vi "GoalieOld.vi"(6 "Defensores":u32[](array[numeric]), 7 "AI Parameters":T1={"GotoKick"={"Dist do cone a frente"=0.0, "attacker farback"=1000.0, "Perto"=300.0, "min dist to kick"=0.0, "kick eps"=110.0, "Time to transition"=0.05}, "Attacker"={"CC chute"=0.09, "CC passe"=0.045, "Kick Force"=200.0, "D ball-robot Kick"=200.0, "D ball-robot Pass"=0.0}, "Defender"={"D max"=1700.0, "Vel p/ robô av"=1000.0, "Kick Force"=100.0, "D atk-def"=300.0, "D farback"=400.0}, "Timeout"={"Field/v in x"=6.0, "Dist Robots"=300, "Dist up in y"=300}, "Pose Striker"={"dist"=200.0, "Numeric"=-4.0, "dist 2"=200.0}, "Dist Stop"=300.0, "Distance when ball out"=200, "D central gap "=150.0, "T pass"=0.0, "Force ++"=0.0, "range kick"=0.0, "Chute alto"=TRUE, "Marcador novo"=TRUE} {"D central gap" format="%#_13g"; "Dist Stop" format="%#_13g"; "Pose Striker"."Numeric" format="%#_13g"; "Defender"."Kick Force" format="%#_13g"; "Defender"."Vel p/ robô av" format="%#_13g"; "Attacker"."D ball-robot Kick" format="%#_13g"; "Attacker"."Kick Force" format="%#_13g"; "Attacker"."CC passe" format="%#_13g"; "Attacker"."CC chute" format="%#_13g"; "GotoKick"."min dist to kick" format="%#_13g"; "GotoKick"."Perto" format="%#_13g"; "GotoKick"."attacker farback" format="%#_13g"; "GotoKick"."Dist do cone a frente" format="%#_13g"}, 8 "Robot":T2={"id"=0, "function"=enum."Attacker", "x"=0.0, "y"=0.0, "orientation"=0.0, "v_tangent"=0.0, "v_normal"=0.0, "v_ang"=0.0, "kick_x"=0.0, "kick_z"=0.0, "dribble"=FALSE, "Timestamp"=timestamp(0 s since 1904-01-01), "estimatives"={"est_v_tangent"=0.0, "est_v_normal"=0.0, "est_vx"=0.0, "est_vy"=0.0, "Pos Robot Est"=[]}, "dest_x_kick"=0.0, "dest_y_kick"=0.0, "Gap Coord"=[], "States"=enum."GoToTangent", "Path "=[], "Path  Smooth"=[], "Dest"=[]}, 10 "Field defense":dbl[](array[numeric]), 11 "IA Input":T7={"our_robots"=[], "enemy_robots"=[], "balls"=[], "geometry"={"line_width"=0, "field_length"=0, "field_width"=0, "boundary_width"=0, "referee_width"=0, "goal_width"=0, "goal_depth"=0, "goal_wall_width"=0, "center_circle_radius"=0, "defense_radius"=0, "defense_stretch"=0, "free_kick_from_defense_dist"=0, "penalty_spot_from_field_line_dist"=0, "penalty_line_from_spot_dist"=0}, "IA Judge"={"stage"="", "command"="", "our_goalie_id"=0.0, "enemy_goalie_id"=0.0, "command enum"=enum."Halt", "Time"=enum."Azul"}, "Received Timestamp"=timestamp(0 s since 1904-01-01), "Events"={"Touch"=FALSE, "Ball out"=FALSE, "id touch"=0.0, "Ball out of \nVision"=FALSE, "Ball inside \nGoalie area"=FALSE, "Robot not responding"=FALSE, "Robots responding status"=[1.0, 1.0, 1.0, 1.0, 1.0, 1.0], "Enemy Ball \nPossession"=FALSE, "Pass State"=FALSE, "id end of pass"=0.0, "Kick"=FALSE, "Id ini Possession"=0.0, "Ball Possesion"=FALSE, "Id Possesion"=0.0}}) -> (2 "output cluster":T2={"id"=0, "function"=enum."Attacker", "x"=0.0, "y"=0.0, "orientation"=0.0, "v_tangent"=0.0, "v_normal"=0.0, "v_ang"=0.0, "kick_x"=0.0, "kick_z"=0.0, "dribble"=FALSE, "Timestamp"=timestamp(0 s since 1904-01-01), "estimatives"={"est_v_tangent"=0.0, "est_v_normal"=0.0, "est_vx"=0.0, "est_vy"=0.0, "Pos Robot Est"=[]}, "dest_x_kick"=0.0, "dest_y_kick"=0.0, "Gap Coord"=[], "States"=enum."GoToTangent", "Path "=[], "Path  Smooth"=[], "Dest"=[]})   [LabVIEW 2017]
uses:
  Core/AI Input.ctl
  Core/AI Robot.ctl
  Functions Enum.ctl
  AttackerStates.ctl
  Path Planning/RRT/PathDests.ctl
  Path Planning/RRT/PathDest.ctl
  Core/AI Ball.ctl
  Core/Field Size.ctl
  Core/AI Judge.ctl
  Command Enum.ctl
  Util/Events/Events.ctl
  AI Parameters.ctl
panel:
  in  "Time kick (s)":dbl=1.0 caption="Time Target (s)"
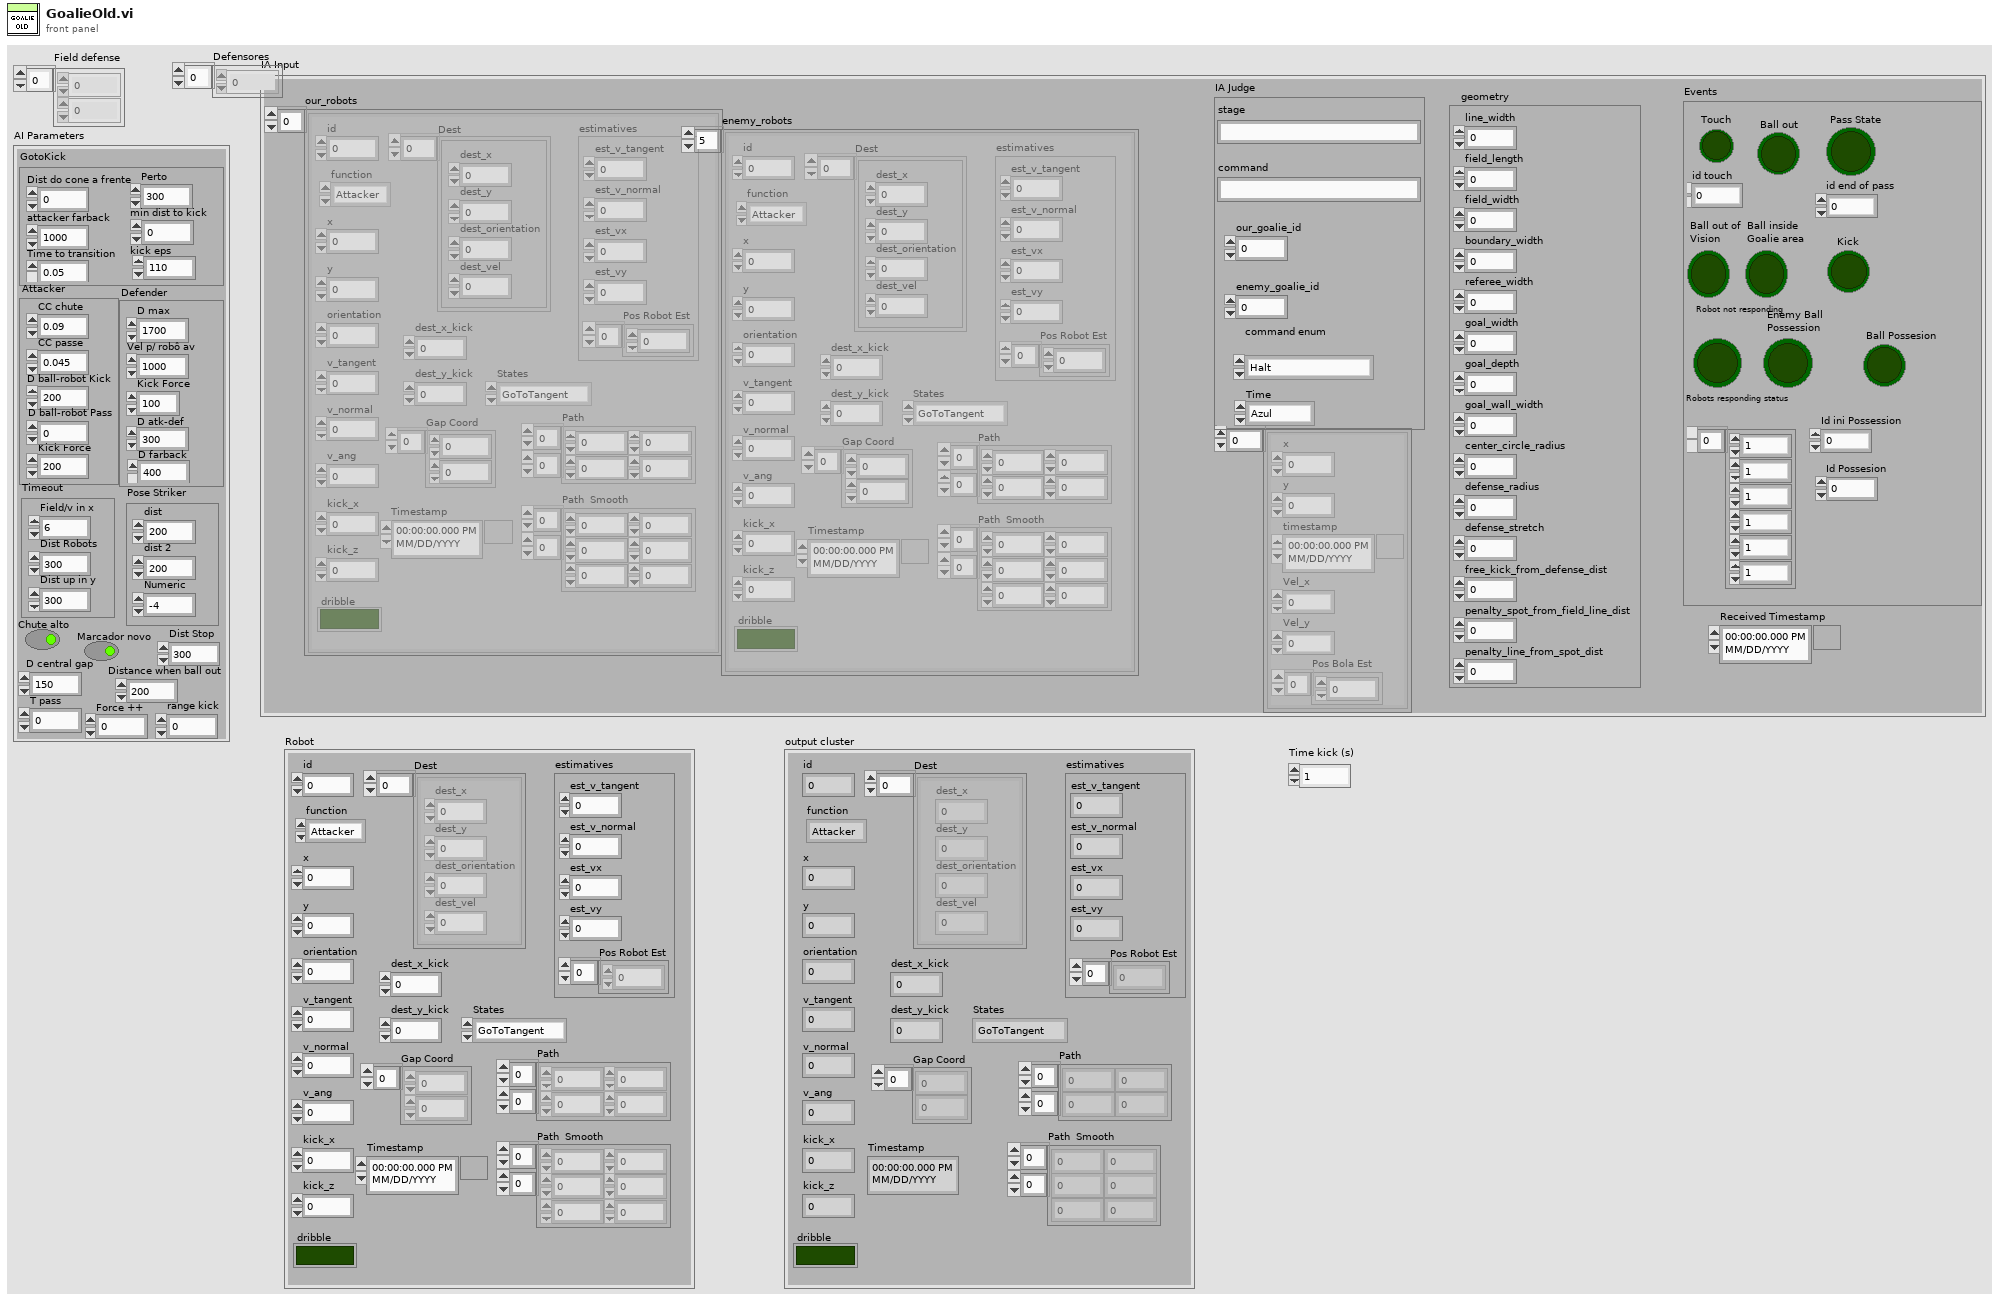
[diagram p1: front panel]
types:
  T1 = typedef "AI Parameters.ctl" = cluster{"GotoKick":cluster{"Dist do cone a frente":dbl, "attacker farback":dbl, "Perto":dbl, "min dist to kick":dbl, "kick eps":dbl, "Time to transition":dbl}, "Attacker":cluster{"CC chute":dbl, "CC passe":dbl, "Kick Force":dbl, "D ball-robot Kick":dbl, "D ball-robot Pass":dbl}, "Defender":cluster{"D max":dbl, "Vel p/ robô av":dbl, "Kick Force":dbl, "D atk-def":dbl, "D farback":dbl}, "Timeout":cluster{"Field/v in x":dbl, "Dist Robots":u32, "Dist up in y":u32}, "Pose Striker":cluster{"dist":dbl, "Numeric":dbl, "dist 2":dbl}, "Dist Stop":dbl, "Distance when ball out":i32, "D central gap ":dbl, "T pass":dbl, "Force ++":dbl, "range kick":dbl, "Chute alto":bool, "Marcador novo":bool}
  T2 = typedef "AI Robot.ctl" = cluster{"id":u32, "function":T3, "x":dbl, "y":dbl, "orientation":dbl, "v_tangent":dbl, "v_normal":dbl, "v_ang":dbl, "kick_x":dbl, "kick_z":dbl, "dribble":bool, "Timestamp":timestamp, "estimatives":cluster{"est_v_tangent":dbl, "est_v_normal":dbl, "est_vx":dbl, "est_vy":dbl, "Pos Robot Est":dbl[]}, "dest_x_kick":dbl, "dest_y_kick":dbl, "Gap Coord":dbl[], "States":T4, "Path ":dbl[][], "Path  Smooth":dbl[][], "Dest":T5}
  T3 = typedef "Functions Enum.ctl" = enum16{"Attacker", "Goalie", "Defender", "Striker", "Goto 0", "Dummy", "Kicker", "ZigZag"}
  T4 = typedef "AttackerStates.ctl" = enum16{"Pass", "GoToTangent", "BallGetting", "GoToKick", ""}
  T5 = typedef "PathDests.ctl" = T6[]
  T6 = typedef "PathDest.ctl" = cluster{"dest_x":dbl, "dest_y":dbl, "dest_orientation":dbl, "dest_vel":dbl}
  T7 = typedef "AI Input.ctl" = cluster{"our_robots":T2[], "enemy_robots":T2[], "balls":T8[], "geometry":T9, "IA Judge":T10, "Received Timestamp":timestamp, "Events":T12}
  T8 = typedef "AI Ball.ctl" = cluster{"x":dbl, "y":dbl, "timestamp":timestamp, "Vel_x":dbl, "Vel_y":dbl, "Pos Bola Est":dbl[]}
  T9 = typedef "Field Size.ctl" = cluster{"line_width":u32, "field_length":u32, "field_width":u32, "boundary_width":u32, "referee_width":u32, "goal_width":u32, "goal_depth":u32, "goal_wall_width":u32, "center_circle_radius":u32, "defense_radius":u32, "defense_stretch":u32, "free_kick_from_defense_dist":u32, "penalty_spot_from_field_line_dist":u32, "penalty_line_from_spot_dist":u32}
  T10 = typedef "AI Judge.ctl" = cluster{"stage":string, "command":string, "our_goalie_id":dbl, "enemy_goalie_id":dbl, "command enum":T11, "Time":enum16{"Azul", "Amarelo"}}
  T11 = typedef "Command Enum.ctl" = enum16{"Halt", "Stop", "Force Start", "PKA Normal Start", "Prepare Kickoff Ally", "PKE Normal Start", "Prepare Kickoff Enemy", "Prepare Penalty Ally", "PPA Normal Start", "Prepare Penalty Enemy", "PPE Normal Start", "Direct Free Enemy", "Direct Free Ally", "Indirect Free Enemy", "Indirect Free Ally", "Timeout Enemy", "Timeout Ally", "Goal Enemy", "Goal Ally", "Ball Placement Enemy", "Ball Placement Ally", "Normal Half Time", "Extra Time Break", "Extra Half Time", "None", "Post Game"}
  T12 = typedef "Events.ctl" = cluster{"Touch":bool, "Ball out":bool, "id touch":dbl, "Ball out of \nVision":bool, "Ball inside \nGoalie area":bool, "Robot not responding":bool, "Robots responding status":dbl[], "Enemy Ball \nPossession":bool, "Pass State":bool, "id end of pass":dbl, "Kick":bool, "Id ini Possession":dbl, "Ball Possesion":bool, "Id Possesion":dbl}
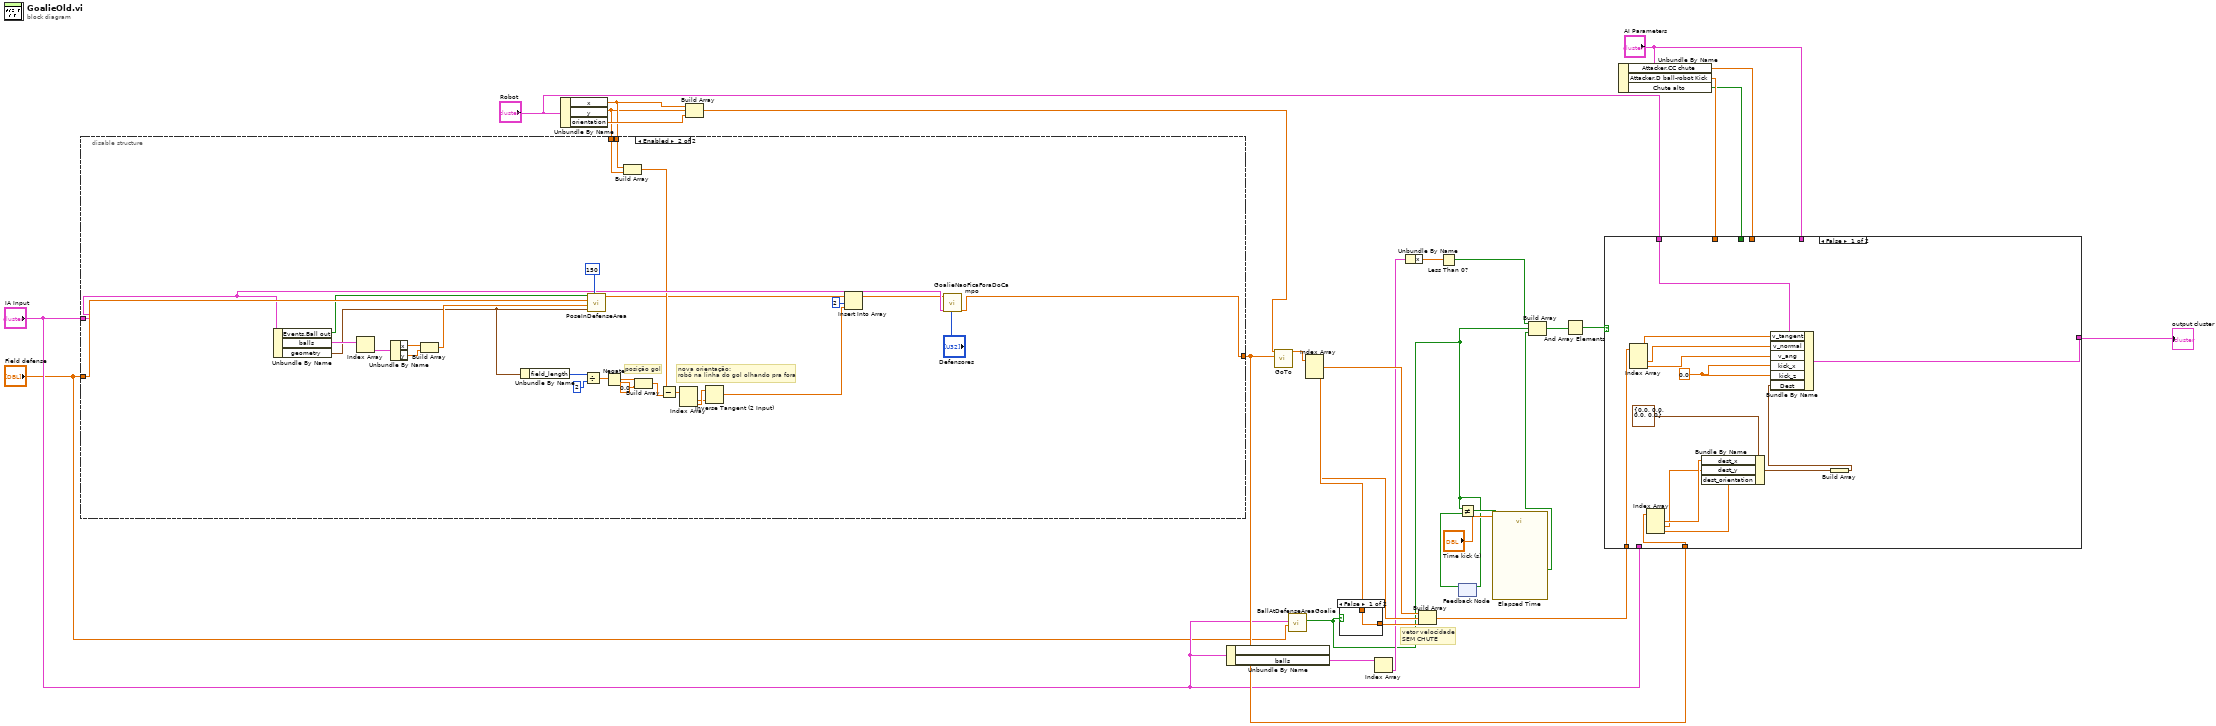
[diagram p0: block diagram]
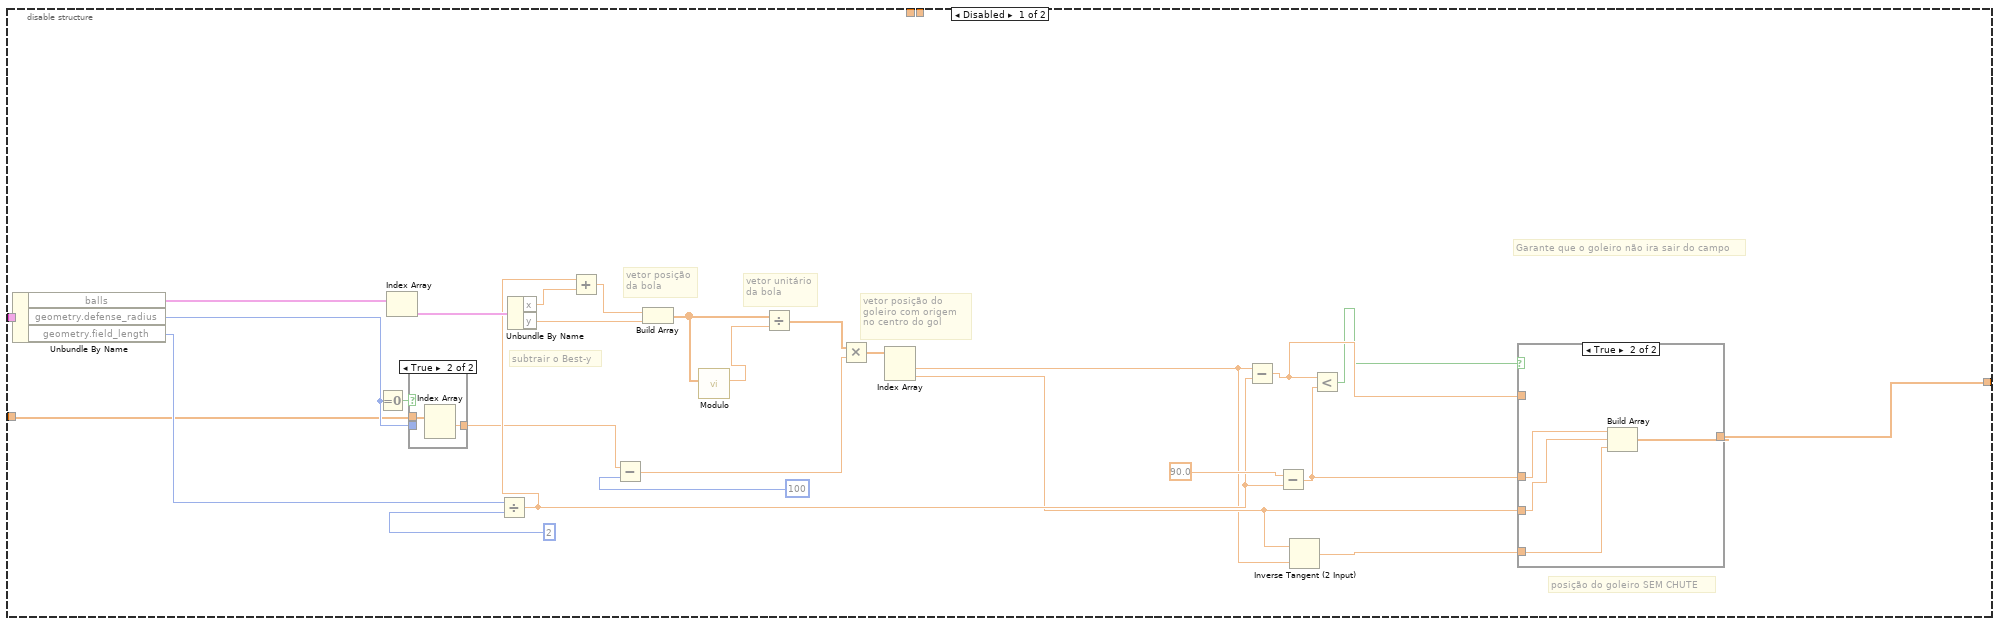
[diagram p2: hidden frame]
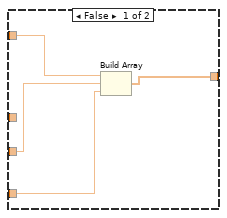
[diagram p4: hidden frame]
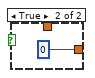
[diagram p5: hidden frame]
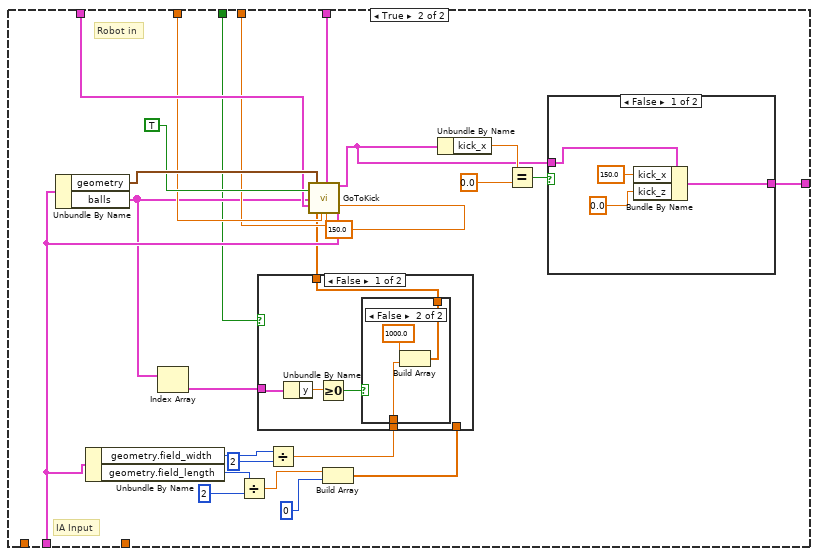
[diagram p6: hidden frame]
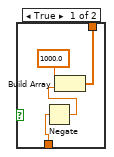
[diagram p7: hidden frame]
diagram:
  # "vetor velocidade SEM CHUTE"
  n1 = Unbundle By Name("Robot") -> ("x"=w8:dbl, "y"=w7:dbl, "orientation"=w30:dbl)
  n2 = disable-structure shown="Enabled" {
    disable-tunnel: "IA Input" -> [w36 w87]
    disable-tunnel: [w35 w88] -> w5
    disable-tunnel: "Field defense" -> [w31 w96]
    disable-tunnel: w8 -> [_ w75]
    disable-tunnel: w7 -> [_ w74]
    frame Disabled {
      # "posição do goleiro SEM CHUTE"
      # "Garante que o goleiro não ira sair do campo"
      # "vetor posição do goleiro com origem no centro do gol"
      # "subtrair o Best-y"
      # "vetor unitário da bola"
      # "vetor posição da bola"
      n3 = Unbundle By Name(w36) -> ("balls"=w57:T8[], "geometry.defense_radius"=w32:u32, "geometry.field_length"=w42:u32)
      n4 = Equal To 0?(x=w32) -> (x = 0?=w33:bool)
      n5 = Index Array(array=w57) -> (element=w56:T8)  [unwired: 1 in]
      n6 = case shown="True" w33 {
        tunnel: [w58 w59] -> w34
        tunnel: w32 -> [w58 _]
        tunnel: w31 -> [_ w60]
        frame False {
        }
        frame True {
          n7 = Index Array(array=w60) -> (element #2=w59:dbl)  [unwired: 2 in, 1 out]
        }
      }
      n8 = Divide(x=w42, y=u32 2) -> (x/y=w41:dbl)
      n9 = Unbundle By Name(w56) -> ("x"=w43:dbl, "y"=w44:dbl)
      n10 = Add(x=w41, y=w43) -> (x+y=w40:dbl)
      n11 = Subtract(x=w34, y=u32 100) -> (x-y=w52:dbl)
      n12 = Build Array(w40, w44) -> (w55:dbl[])
      n13 = call "Modulo.vi"("2D vector"=w55) -> ("Modulo"=w54:dbl)  [unwired: 10 in]
      n14 = Divide(x=w55, y=w54) -> (x/y=w53:dbl[])
      n15 = Multiply(x=w53, y=w52) -> (x*y=w50:dbl[])
      n16 = Index Array(array=w50) -> (element #1=w38:dbl, element #2=w39:dbl)  [unwired: 2 in]
      n17 = Subtract(x=w38, y=w41) -> (x-y=w46:dbl)
      n18 = Subtract(x=90.0, y=w41) -> (x-y=w47:dbl)
      n19 = Inverse Tangent (2 Input)(1:w38, 2:w39) -> (0:w37:dbl)
      n20 = Less?(x=w46, y=w47) -> (x < y?=w45:bool)
      n21 = case shown="True" w45 {
        tunnel: w39 -> [w63 w66]
        tunnel: w47 -> [_ w68]
        tunnel: w46 -> [w64 _]
        tunnel: [w62 w67] -> w35
        tunnel: w37 -> [w61 w65]
        frame False {
          n22 = Build Array(w64, w63, w61) -> (w62:dbl[])
        }
        frame True {
          n23 = Build Array(w68, w66, w65) -> (w67:dbl[])
        }
      }
    }
    frame Enabled {
      # "nova orientação:\nrobô na linha do gol olhando pra fora"
      # "posição gol"
      n24 = Unbundle By Name(w87) -> ("Events.Ball out"=w89:bool, "balls"=w91:T8[], "geometry"=w76:T9)
      n25 = Index Array(array=w91) -> (element=w92:T8)  [unwired: 1 in]
      n26 = Unbundle By Name(w92) -> ("x"=w93:dbl, "y"=w94:dbl)
      n27 = Build Array(w93, w94) -> (w90:dbl[])
      n28 = Unbundle By Name(w76) -> ("field_length"=w85:u32)
      n29 = Divide(x=w85, y=u32 2) -> (x/y=w83:dbl)
      n30 = call "PoseInDefenseArea.vi"("Recuo"=u32 150, "geometry"=w76, "Ball"=w90, "Field defense"=w96, "Events.Ball out"=w89) -> ("Array"=w72:dbl[])  [unwired: 6 in]
      n31 = Negate(x=w83) -> (-x=w82:dbl)
      n32 = Build Array(w75, w74) -> (w73:dbl[])
      n33 = Build Array(w82, 0.0 ("element")) -> (w80:dbl[])
      n34 = Subtract(x=w73, y=w80) -> (x-y=w79:dbl[])
      n35 = Index Array(array=w79) -> (element #1=w77:dbl, element #2=w78:dbl)  [unwired: 2 in]
      n36 = Inverse Tangent (2 Input)(1:w77, 2:w78) -> (0:w70:dbl)
      n37 = Insert Into Array(array=w72, index=2, new element=w70) -> (w69:dbl[])
      n38 = call "GoalieNaoFicaForaDoCampo.vi"("Defensores"="Defensores", "IA Input"=w87, "PositionIn"=w69) -> ("PositionOut"=w88:dbl[])  [unwired: 8 in]
    }
  }
  n39 = Build Array(w8, w7, w30) -> (w29:dbl[])
  n40 = Unbundle By Name("IA Input") -> ("balls"=w14:T8[])  [unwired: 1 out]
  n41 = call "GoTo.vi"("Target"=w5, "Position"=w29) -> ("Output\nVelocity"=w28:dbl[])  [unwired: 8 in, 1 out]
  n42 = call "BallAtDefenseAreaGoalie.vi"("Field defense"="Field defense", "IA State"="IA Input") -> ("Ball at goalkeeper area ?"=w2:bool)  [unwired: 9 in]
  n43 = Index Array(array=w28) -> (element #1=w23:dbl, element #2=w24:dbl, element #3=w25:dbl)  [unwired: 3 in]
  n44 = case shown="False" w2 {
    tunnel: [w97 0] -> w26
    tunnel: w25 -> [w97 _]
    frame False {
    }
    frame True {
    }
  }
  n45 = Index Array(array=w14) -> (element=w13:T8)  [unwired: 1 in]
  n46 = Unbundle By Name(w13) -> ("x"=w12:dbl)
  n47 = Build Array(w23, w24, w26) -> (w21:dbl[])
  n48 = Less Than 0?(x=w12) -> (x < 0?=w11:bool)
  n49 = feedback #1() -> (w17:bool)  [unwired: 1 in]
  n50 = feedback-in #1(w2) -> ()
  n51 = Not Equal?(x=w2, y=w17) -> (x != y?=w19:bool)
  n52 = call "Elapsed Time"("Time Target (s)"="Time kick (s)", "Reset"=w19) -> ("Time has Elapsed"=w18:bool)  [unwired: 10 in, 7 out]
  n53 = Build Array(w11, w2, w18) -> (w15:bool[])
  n54 = And Array Elements(Boolean array=w15) -> (logical AND=w16:bool)
  n55 = Unbundle By Name("AI Parameters") -> ("Attacker.CC chute"=w9:dbl, "Attacker.D ball-robot Kick"=w10:dbl, "Chute alto"=w1:bool)
  n56 = case shown="False" w16 {
    tunnel: "IA Input" -> [_ w133]
    tunnel: "Robot" -> [w112 w135]
    tunnel: [w111 w122] -> w22
    tunnel: w21 -> [w109 _]
    tunnel: w5 -> [w105 _]
    tunnel: "AI Parameters" -> [_ w128]
    tunnel: w10 -> [_ w127]
    tunnel: w9 -> [_ w126]
    tunnel: w1 -> [_ w113]
    frame False {
      w110 = 0.0 ("kick_z")
      n57 = Index Array(array=w109) -> (element #1=w108:dbl, element #2=w107:dbl, element #3=w106:dbl)  [unwired: 3 in]
      n58 = Index Array(array=w105) -> (element #1=w102:dbl, element #2=w101:dbl, element #3=w100:dbl)  [unwired: 3 in]
      n59 = Bundle By Name(cluster=T6 {"dest_x"=0.0, "dest_y"=0.0, "dest_orientation"=0.0, "dest_vel"=0.0} ("element"), "dest_x"=w102, "dest_y"=w101, "dest_orientation"=w100) -> (w103:T6)
      n60 = Build Array(w103) -> (w99:T6[])
      n61 = Bundle By Name(cluster=w112, "v_tangent"=w108, "v_normal"=w107, "v_ang"=w106, "kick_x"=w110, "kick_z"=w110, "Dest"=w99) -> (w111:T2)
    }
    frame True {
      # "Robot in"
      # "IA Input"
      n62 = Unbundle By Name(w133) -> ("geometry"=w137:T9, "balls"=w118:T8[])
      n63 = Unbundle By Name(w133) -> ("geometry.field_width"=w115:u32, "geometry.field_length"=w132:u32)
      n64 = Index Array(array=w118) -> (element=w117:T8)  [unwired: 1 in]
      n65 = Divide(x=w132, y=u32 2) -> (x/y=w130:dbl)
      n66 = Divide(x=w115, y=u32 2) -> (x/y=w114:dbl)
      n67 = Build Array(w130, 0) -> (w119:dbl[])
      n68 = case shown="False" w113 {
        tunnel: [w139 w150] -> w120
        tunnel: w119 -> [_ w150]
        tunnel: w117 -> [w142 _]
        tunnel: w114 -> [w138 _]
        frame False {
          n69 = Unbundle By Name(w142) -> ("y"=w141:dbl)
          n70 = Greater Or Equal To 0?(x=w141) -> (x >= 0?=w140:bool)
          n71 = case shown="False" w140 {
            tunnel: [w146 w149] -> w139
            tunnel: w138 -> [w144 w147]
            frame True {
              n72 = Negate(x=w144) -> (-x=w143:dbl)
              n73 = Build Array(1000.0 ("element"), w143) -> (w146:dbl[])
            }
            frame False {
              n74 = Build Array(1000.0 ("element"), w147) -> (w149:dbl[])
            }
          }
        }
        frame True {
        }
      }
      n75 = call "GoToKick.vi"("goleiro?"=TRUE, "balls"=w118, "Robot in in"=w135, "Field Size in"=w137, "Target"=w120, "D ball - robot"=w127, "AI Parameters"=w128, "Cone de chute"=w126, "Kick Force"=150.0, "IA State Input in"=w133) -> ("Robot out"=w121:T2)  [unwired: 6 in, 3 out]
      n76 = Unbundle By Name(w121) -> ("kick_x"=w123:dbl)
      n77 = Equal?(x=w123, y=0.0) -> (x = y?=w125:bool)
      n78 = case shown="False" w125 {
        tunnel: [w152 w155] -> w122
        tunnel: w121 -> [w154 w155]
        frame False {
          n79 = Bundle By Name(cluster=w154, "kick_x"=150.0, "kick_z"=0.0) -> (w152:T2)
        }
        frame True {
        }
      }
    }
  }
  "output cluster" <- w22
